vi "生成product表头.vi"() -> (3 "product信息":T1)   [LabVIEW 2017]
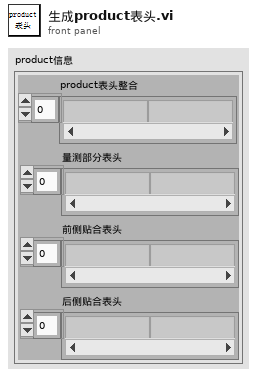
[diagram p1: front panel]
types:
  T1 = typedef "product信息.ctl" = cluster{"product表头整合":string[], "量测部分表头":string[], "前侧贴合表头":string[], "后侧贴合表头":string[]}
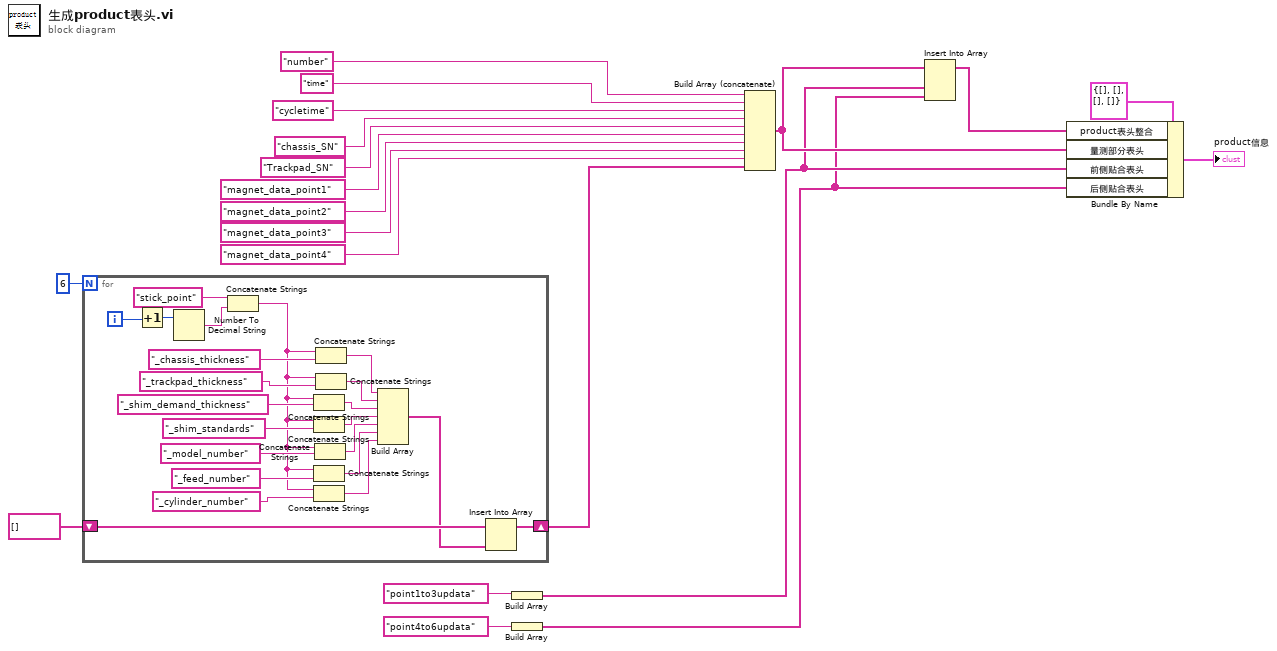
[diagram p0: block diagram]
diagram:
  n1 = for {
    N: 6 -> [_]
    shift-right: [w28] -> w12
    shift-left: string[] [] -> [w29]
    i -> [w42]
    n2 = Increment(x=w42) -> (x+1=w41:i32)
    n3 = Number To Decimal String(number=w41) -> (decimal integer string=w39:string)  [unwired: 1 in]
    n4 = Concatenate Strings("stick_point", w39) -> (w25:string)
    n5 = Concatenate Strings(w25, "_shim_demand_thickness") -> (w30:string)
    n6 = Concatenate Strings(w25, "_shim_standards") -> (w24:string)
    n7 = Concatenate Strings(w25, "_feed_number") -> (w22:string)
    n8 = Concatenate Strings(w25, "_cylinder_number") -> (w21:string)
    n9 = Concatenate Strings(w25, "_model_number") -> (w23:string)
    n10 = Concatenate Strings(w25, "_chassis_thickness") -> (w32:string)
    n11 = Concatenate Strings(w25, "_trackpad_thickness") -> (w31:string)
    n12 = Build Array(w32, w31, w30, w24, w23, w22, w21) -> (w27:string[])
    n13 = Insert Into Array(array=w29, new element=w27) -> (w28:string[])  [unwired: 1 in]
  }
  n14 = Build Array("point1to3updata") -> (w4:string[])
  n15 = Build Array("point4to6updata") -> (w1:string[])
  n16 = Build Array (concatenate)("number", "time", "cycletime", "chassis_SN", "Trackpad_SN", "magnet_data_point1", "magnet_data_point2", "magnet_data_point3", "magnet_data_point4", w12) -> (w5:string[])
  n17 = Insert Into Array(array=w5, new element #1=w4, new element #2=w1) -> (w3:string[])  [unwired: 1 in]
  n18 = Bundle By Name(cluster=T1 {"product表头整合"=[], "量测部分表头"=[], "前侧贴合表头"=[], "后侧贴合表头"=[]} ("product信息"), "product表头整合"=w3, "量测部分表头"=w5, "前侧贴合表头"=w4, "后侧贴合表头"=w1) -> (→"product信息":T1)
